vi "Exposure-Options Dialog.vi"(10 "Tracking":T1={"Tracking"={"Tolerance (dB)"=0.25, "T (s)"=3.0}, "Seeds"={"Left"=0, "Right"=0}}) -> (2 "Tracking out":T1={"Tracking"={"Tolerance (dB)"=0.25, "T (s)"=3.0}, "Seeds"={"Left"=0, "Right"=0}}, 3 "Cancelled?":bool=TRUE)   [LabVIEW 2020]
doc: "Use this template to create a dialog box with event handling."
uses:
  Typedefs/Exposure-Options.ctl
panel:
  in  "Right":i32
  in  "Left":i32
  in  "Time (s)":dbl
  in  "Tolerance (dB)":dbl
  in  "Cancel":bool
  in  "OK":bool
  # "Level Tracking"
  # "Noise seeds"
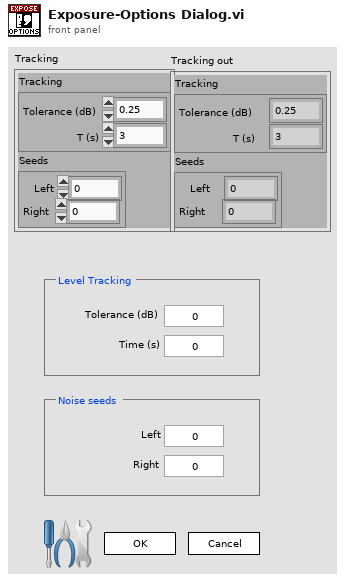
[diagram p1: front panel]
types:
  T1 = typedef "Exposure-Options.ctl" = cluster{"Tracking":cluster{"Tolerance (dB)":dbl, "T (s)":dbl}, "Seeds":cluster{"Left":i32, "Right":i32}}
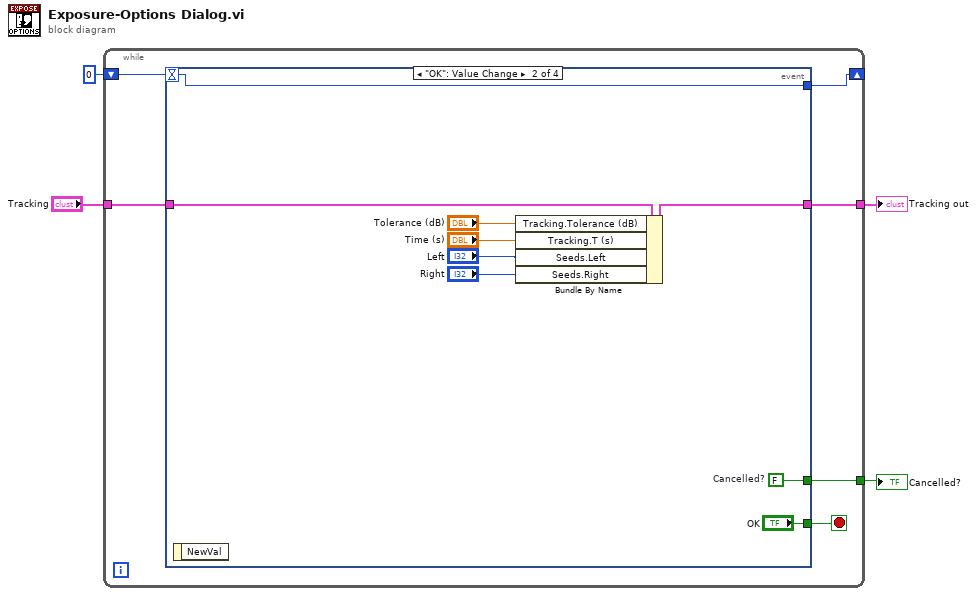
[diagram p0: block diagram]
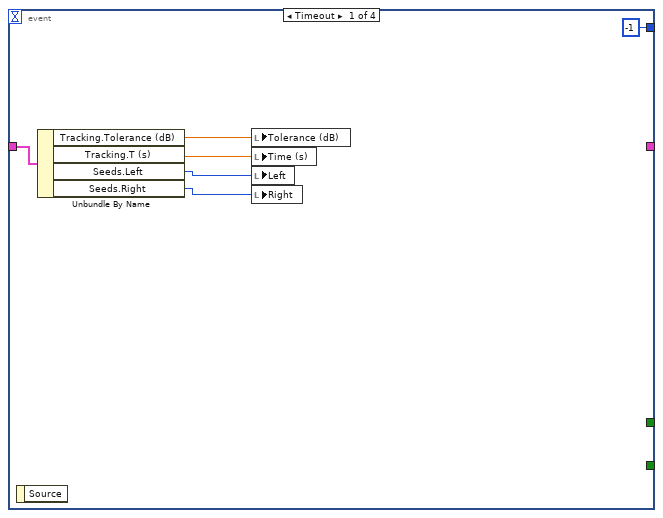
[diagram p2: hidden frame]
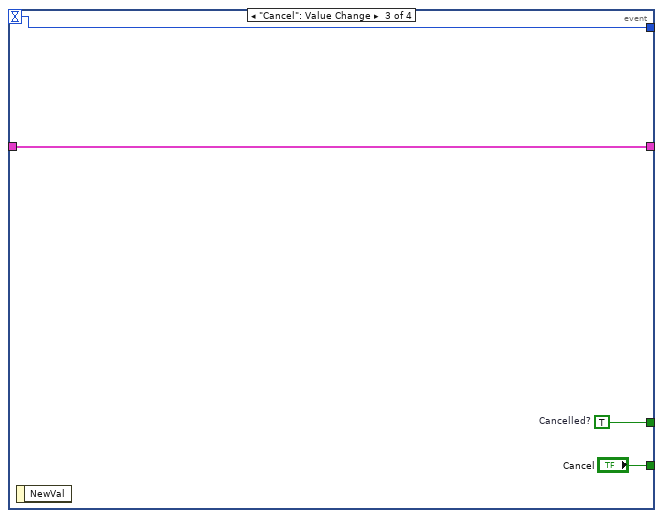
[diagram p3: hidden frame]
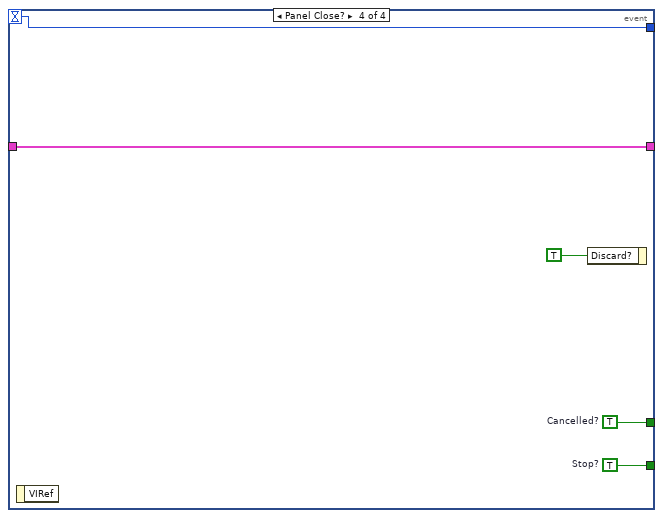
[diagram p4: hidden frame]
diagram:
  n1 = while {
    tunnel: [w9] -> w4
    shift-right: [w7] -> _
    shift-left: 0 -> [w8]
    tunnel: "Tracking" -> [w6]
    tunnel: [w5] -> w1
    stop <- w10 stop-if-true
    n2 = event shown="[1] \"OK\": Value Change" {
      selector: _ -> [_ _ _ _]
      dyn-events: _ -> [_ _ _ _]
      timeout: w8 -> [_ w23 w27 w31]
      tunnel: [_ "OK" "Cancel" w33] -> w10
      tunnel: [_ w25 w29 w32] -> w9
      tunnel: [-1 w23 w27 w31] -> w7
      tunnel: w6 -> [w15 w22 w26 w30]
      tunnel: [_ w20 w26 w30] -> w5
      event Timeout {
        n3 = event-data() -> ()  [unwired: 1 in, 1 out]
        n4 = Unbundle By Name(w15) -> ("Tracking.Tolerance (dB)"=w14:dbl, "Tracking.T (s)"=w13:dbl, "Seeds.Left"=w12:i32, "Seeds.Right"=w11:i32)
        n5 = local write "Tolerance (dB)"(w14) -> ()
        n6 = local write "Time (s)"(w13) -> ()
        n7 = local write "Left"(w12) -> ()
        n8 = local write "Right"(w11) -> ()
      }
      event "OK": Value Change {
        w25 = FALSE  # Cancelled?
        n9 = event-data() -> ()  [unwired: 1 in, 1 out]
        n10 = Bundle By Name(cluster=w22, "Tracking.Tolerance (dB)"="Tolerance (dB)", "Tracking.T (s)"="Time (s)", "Seeds.Left"="Left", "Seeds.Right"="Right") -> (w20:T1)
      }
      event "Cancel": Value Change {
        w29 = TRUE  # Cancelled?
        n11 = event-data() -> ()  [unwired: 1 in, 1 out]
      }
      event Panel Close? {
        w32 = TRUE  # Cancelled?
        w33 = TRUE  # Stop?
        n12 = event-data() -> ()  [unwired: 1 in, 1 out]
        n13 = event-data("Discard?"=TRUE) -> ()  [unwired: 1 in, 1 out]
      }
    }
  }
  "Cancelled?" <- w4
  "Tracking out" <- w1
